vi "sub_SDR_mimo_RemovePilots.vi"(8 "Symbols per pilot":i32, 9 "Payload Symbols":i32, 10 "Array in":cdb[](array[numeric])) -> (0 "SNR 2 (dB)":dbl, 1 "SNR 1 (dB)":dbl, 2 "Array Out":cdb[](array[numeric]))   [LabVIEW 2012]
uses:
  <vilib>/Analysis/NI_AALBase.lvlib
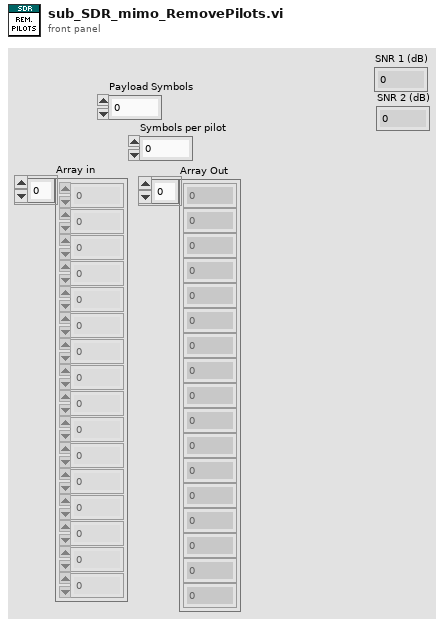
[diagram p1: front panel]
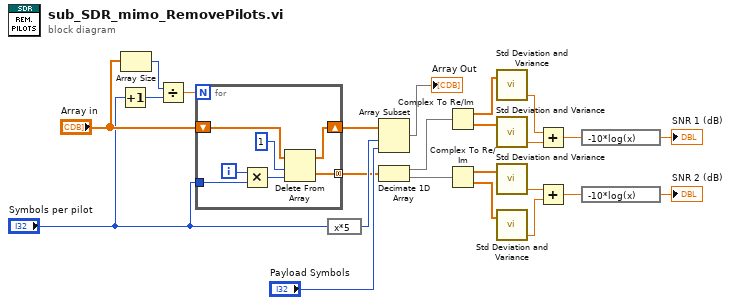
[diagram p0: block diagram]
diagram:
  n1 = Increment(x="Symbols per pilot") -> (x+1=w17:i32)
  n2 = Array Size(array="Array in") -> (size(s)=w20:i32)
  n3 = Divide(x=w20, y=w17) -> (x/y=w21:dbl)
  n4 = for {
    N: w21 -> [_]
    shift-right: [w30] -> w19
    shift-left: "Array in" -> [w31]
    tunnel: "Symbols per pilot" -> [w26]
    tunnel: [w25] -> w15 mode=concatenating
    i -> [w28]
    n5 = Multiply(x=w28, y=w26) -> (x*y=w27:i32)
    n6 = Delete From Array(array=w31, length=1, index=w27) -> (deleted portion=w25:cdb[], array with subset deleted=w30:cdb[])
  }
  n7 = expression code="x*5"("Symbols per pilot") -> (w24:i32)
  n8 = Array Subset(array=w19, index=w24, length="Payload Symbols") -> (→"Array Out":cdb[])
  n9 = Decimate 1D Array(w15) -> (w3:cdb[], w2:cdb[])
  n10 = Complex To Re/Im(x + iy=w3) -> (x=w14:dbl[], y=w13:dbl[])
  n11 = Complex To Re/Im(x + iy=w2) -> (x=w8:dbl[], y=w7:dbl[])
  n12 = call <vilib>:"Std Deviation and Variance.vi"("X"=w14) -> ("variance"=w12:dbl)  [unwired: 1 in, 2 out]
  n13 = call <vilib>:"Std Deviation and Variance.vi"("X"=w13) -> ("variance"=w11:dbl)  [unwired: 1 in, 2 out]
  n14 = call <vilib>:"Std Deviation and Variance.vi"("X"=w8) -> ("variance"=w6:dbl)  [unwired: 1 in, 2 out]
  n15 = call <vilib>:"Std Deviation and Variance.vi"("X"=w7) -> ("variance"=w5:dbl)  [unwired: 1 in, 2 out]
  n16 = Add(x=w12, y=w11) -> (x+y=w9:dbl)
  n17 = Add(x=w6, y=w5) -> (x+y=w1:dbl)
  n18 = expression code="-10*log(x)"(w9) -> (→"SNR 1 (dB)":dbl)
  n19 = expression code="-10*log(x)"(w1) -> (→"SNR 2 (dB)":dbl)
